vi "Wait for event.vi"(8 "error in (no error)":errorcluster, 10 "String":string, 11 "Notifier in":refnum<notifier>) -> (0 "error out":errorcluster, 3 "Notifier out":refnum<notifier>)   [LabVIEW 2014]
panel:
  # "LICENSED MATERIALS – PROPERTY OF IBM\nCopyright IBM Corp. 2016,\nALL RIGHTS RESERVED"
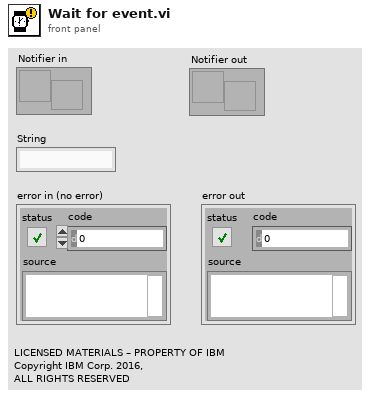
[diagram p1: front panel]
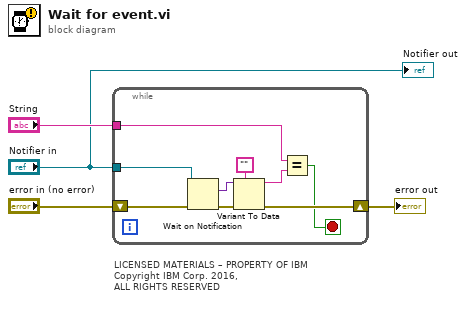
[diagram p0: block diagram]
diagram:
  # "LICENSED MATERIALS – PROPERTY OF IBM\nCopyright IBM Corp. 2016,\nALL RIGHTS RESERVED"
  n1 = while {
    shift-right: [w11] -> w4
    shift-left: "error in (no error)" -> [w13]
    tunnel: "Notifier in" -> [w6]
    tunnel: "String" -> [w5]
    stop <- w7 stop-if-true
    n2 = Wait on Notification(notifier=w6, error in (no error)=w13) -> (notification=w9:variant, error out=w12:errorcluster)  [unwired: 4 out]
    n3 = Variant To Data(error in=w12, type="", Variant=w9) -> (data=w8:string, error out=w11:errorcluster)
    n4 = Equal?(x=w5, y=w8) -> (x = y?=w7:bool)
  }
  "error out" <- w4
  "Notifier out" <- "Notifier in"
